vi "Serial Loopback Interrupt (Host).vi"() -> ()   [LabVIEW 2022 SP3]
doc: "This is the top level VI for a cRIO target. This example will perform a read and a write from the same port on the 987x module. You can use this VI to verify that the port is working correctly. This example uses a nested interrupt scheme to send individual bytes to the FPGA VI.\n\nPlease see the block diagram for more detailed comments."
uses:
  <vilib>/rvi/interface/nirviMethod/nirviMethod.xnode
  <vilib>/rvi/interface/nirviOpenFPGA/nirviOpenFPGA.xnode
  <vilib>/rvi/interface/nirviCloseFPGA/nirviCloseFPGA.xnode
  INT FPGA Reference.ctl
  Program Files (x86)/National Instruments/LabVIEW 2022/examples/CompactRIO/Module Specific/NI 987x/Serial Loopback/VIs/9870 Interface Interrupt (FPGA).vi
  FPGA Bitfiles/ni-987xserialloo_FPGATarget2_9870InterfaceInt_BeCryR9q6UY.lvbitx
  <vilib>/FPGAPlugInAG/cRIO-9040/niLvFpga_Open_cRIO-9040.vi
  <vilib>/FPGAPlugInAG/cRIO-9040/niLvFpga_Reset_cRIO-9040.vi
  <vilib>/FPGAPlugInAG/cRIO-9040/niLvFpga_Run_cRIO-9040.vi
  <vilib>/rvi/interface/nirviMethod/StockFPGA_InlinedMethodWaitForSingleIRQ.vi
  <vilib>/FPGAPlugInAG/cRIO-9040/niLvFpga_WaitOnIrq_cRIO-9040.vi
  <vilib>/FPGAPlugInAG/cRIO-9040/niLvFpga_Close_cRIO-9040.vi
panel:
  out "error out":errorcluster
  in  "Byte Timeout":i32=500
  out "Bytes Written":u32
  in  "Bytes to Read":i32=64
  out "Bytes Received":u32
  out "Receive String":string
  in  "Send String":string="ABCDEFGHIJKLMNOPQRSTUVWXYZ-abcdefghijklmnopqrstuvwxyz-0123456789"
  # "Transmit"
  # "Receive"
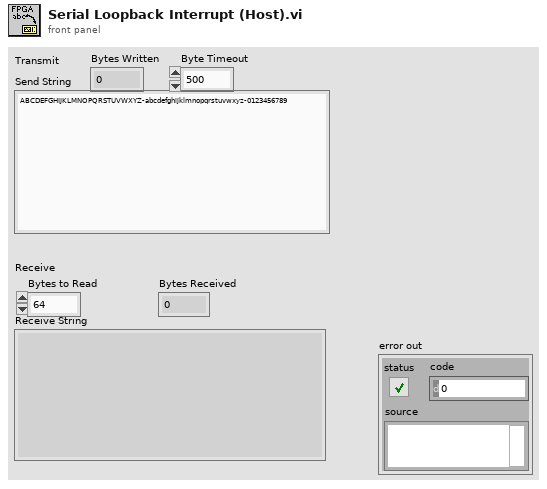
[diagram p1: front panel]
types:
  T1 = typedef "INT FPGA Reference.ctl" = refnum<k20>
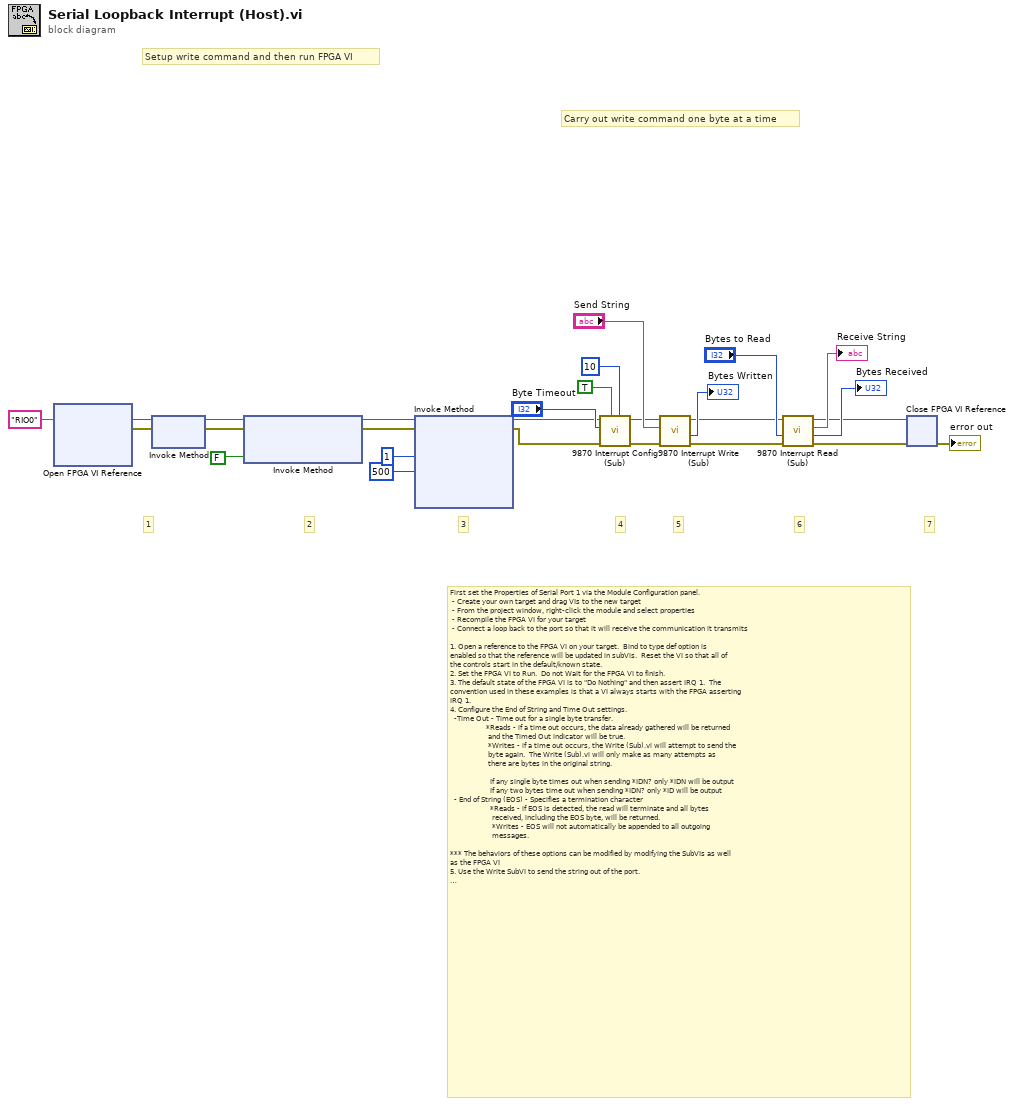
[diagram p0: block diagram]
diagram:
  # "7"
  # "2"
  # "1"
  # "First set the Properties of Serial Port 1 via the Module Configuration panel.\n - Create your own target and drag VIs to the new target\n - From the project window, right-click the module and select properties\n - Recompile the FPGA VI for your target\n - Connect a loop back to the port so that it will receive the communication it transmits\n\n1. Open a reference to the FPGA VI on your target.  Bind to type def option is \nenabled so that the reference will be updated in subVis.  Reset the VI so that all of \nthe controls start in the default/known state.\n2. Set the FPGA VI to Run.  Do not Wait for the FPGA VI to finish.\n3. The default state of the FPGA VI is to \"Do Nothing\" and then assert IRQ 1.  The \nconvention used in these examples is that a VI always starts with the FPGA asserting\nIRQ 1.\n4. Configure the End of String and Time Out settings.  \n  -Time Out - Time out for a single byte transfer.\n                  *Reads - if a time out occurs, the data already gathered will be returned\n                   and the Timed Out indicator will be true.\n                   *Writes - if a time out occurs, the Write (Sub).vi will attempt to send the \n                   byte again.  The Write (Sub).vi will only make as many attempts as \n                   there are bytes in the original string.\n                   \n                    If any single byte times out when sending *IDN? only *IDN will be output\n                    If any two bytes time out when sending *IDN? only *ID will be output\n  - End of String (EOS) - Specifies a termination character\n                    *Reads - if EOS is detected, the read will terminate and all bytes \n                     received, including the EOS byte, will be returned.\n                     *Writes - EOS will not automatically be appended to all outgoing \n                     messages.  \n\n*** The behaviors of these options can be modified by modifying the SubVIs as well\nas the FPGA VI\n5. Use the Write SubVI to send the string out of the port.\n6. Use the Read SubVI to read the data returned to the port.\n7. Close the FPGA VI reference and display any errors"
  # "6"
  # "5"
  # "4"
  # "3"
  # "Carry out write command one byte at a time"
  # "Setup write command and then run FPGA VI"
  n1 = xnode "Open FPGA VI Reference"("resource name"="RIO0") -> ("FPGA VI Reference Out"=w11:T1, "error out"=w26:errorcluster)  [unwired: 1 in]
  n2 = xnode "Invoke Method"("FPGA VI Reference In"=w11, "error in"=w26) -> ("FPGA VI Reference Out"=w10:T1, "error out"=w24:errorcluster)
  n3 = xnode "Invoke Method"("FPGA VI Reference In"=w10, "error in"=w24, "Wait Until Done (F)"=FALSE) -> ("FPGA VI Reference Out"=w7:T1, "error out"=w2:errorcluster)
  n4 = xnode "Invoke Method"("FPGA VI Reference In"=w7, "error in"=w2, "IRQ Number(s)"=1, "Timeout (ms)"=500) -> ("FPGA VI Reference Out"=w4:T1, "error out"=w3:errorcluster)  [unwired: 2 out]
  n5 = call "9870 Interrupt Config (Sub).vi"("EOS Byte"=u8 10, "Enable EOS"=TRUE, "error in"=w3, "Byte Timeout"="Byte Timeout", "FPGA In"=w4) -> ("error out"=w18:errorcluster, "FPGA Out"=w16:T1)  [unwired: 1 in, 4 out]
  n6 = call "9870 Interrupt Write (Sub).vi"("error in"=w18, "Data"="Send String", "FPGA In"=w16) -> ("error out"=w19:errorcluster, "Byte Count"=→"Bytes Written":u32, "FPGA Out"=w12:T1)  [unwired: 1 in, 5 out]
  n7 = call "9870 Interrupt Read (Sub).vi"("error in"=w19, "Number of bytes"="Bytes to Read", "FPGA In"=w12) -> ("error out"=w23:errorcluster, "Byte Count"=→"Bytes Received":u32, "Read Bytes"=→"Receive String":string, "FPGA Out"=w9:T1)  [unwired: 1 in, 4 out]
  n8 = xnode "Close FPGA VI Reference"("FPGA VI Reference In"=w9, "error in"=w23) -> ("error out"=→"error out":errorcluster)
